vi "addTimestampElement.vi"(7 "Name":string, 8 "error in (no error)":errorcluster, 9 "Value":timestamp, 10 "Replace? (false)":bool, 11 "tBSONDocument in":refnum<class "tBSONDocument.lvclass">) -> (0 "error out":errorcluster, 3 "tBSONDocument out":refnum<class "tBSONDocument.lvclass">)   [LabVIEW 2013, in "BSON.lvlib" / "tBSONDocument.lvclass"]
doc: "Adds a timestamp to a BSON document."
uses:
  tBSONDocument.lvclass
  BSONElements/tBSONTimestamp/tBSONTimestamp.lvclass
  tBSONElement/tBSONElement.lvclass
  tBSONElement/setName.vi
  BSONElements/tBSONTimestamp/setValue.vi
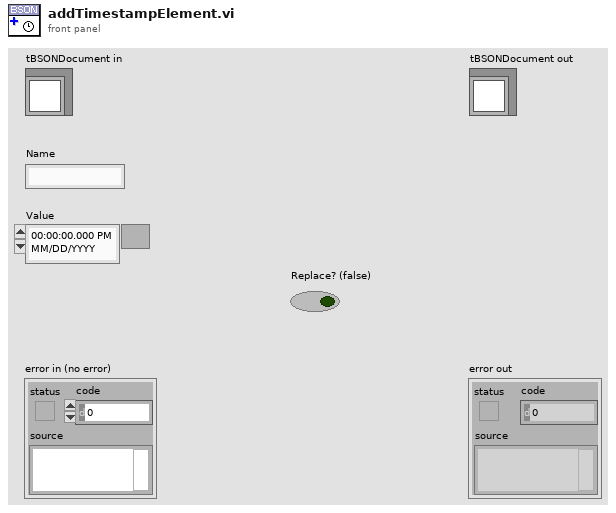
[diagram p1: front panel]
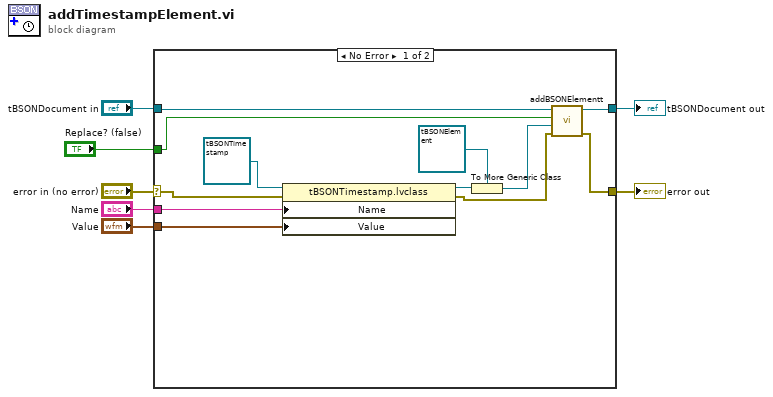
[diagram p0: block diagram]
diagram:
  n1 = case shown="No Error" "error in (no error)" {
    selector: "error in (no error)" -> [w18 w21]
    tunnel: [w9 w21] -> w6
    tunnel: [w12 w20] -> w4
    tunnel: "tBSONDocument in" -> [w13 w20]
    tunnel: "Value" -> [w17 _]
    tunnel: "Name" -> [w16 _]
    tunnel: "Replace? (false)" -> [w8 _]
    frame No Error {
      n2 = property class="tBSONTimestamp.lvclass"(reference=refnum<class "tBSONTimestamp.lvclass"> refnum ("BSON.lvlib:tBSONTimestamp.lvclass"), error in=w18, "Name"=w16, "Value"=w17) -> (reference out=w15:refnum<class "tBSONTimestamp.lvclass">, error out=w10:errorcluster)
      n3 = To More Generic Class(target class=refnum<class "tBSONElement.lvclass"> refnum ("BSON.lvlib:tBSONElement.lvclass"), reference=w15) -> (generic class reference=w11:refnum<class "tBSONElement.lvclass">)
      n4 = call "addBSONElementt.vi"("error in (no error)"=w10, "Element"=w11, "Replace? (false)"=w8, "tBSONDocument in"=w13) -> ("error out"=w9:errorcluster, "tBSONDocument out"=w12:refnum<class "tBSONDocument.lvclass">)  [unwired: 6 in]
    }
    frame Error {
    }
  }
  "error out" <- w6
  "tBSONDocument out" <- w4
